vi "spiral scan.vi"(10 "maximum frequency":dbl, 11 "scan specification":T1) -> (0 "y":i16[](array[numeric]), 1 "x":i16[](array[numeric]), 2 "scan locations":u32[](array[numeric]), 3 "scan specification out":T1)   [LabVIEW 2010]
uses:
  scan_specification_tagResonant.ctl
  <vilib>/Analysis/NI_AALBase.lvlib
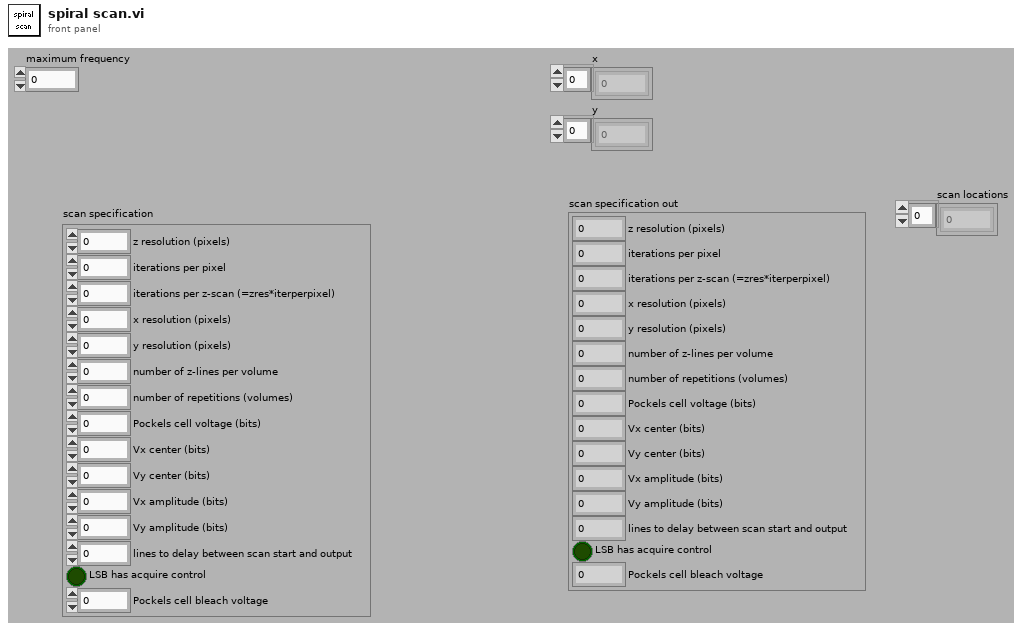
[diagram p1: front panel]
types:
  T1 = typedef "scan_specification_tagResonant.ctl" = cluster{"z resolution (pixels)":u16, "iterations per pixel":u16, "iterations per z-scan (=zres*iterperpixel)":u16, "x resolution (pixels)":u16, "y resolution (pixels)":u16, "number of z-lines per volume":u16, "number of repetitions (volumes)":i32, "Pockels cell voltage (bits)":i16, "Vx center (bits)":i16, "Vy center (bits)":i16, "Vx amplitude (bits)":i16, "Vy amplitude (bits)":i16, "lines to delay between scan start and output":u16, "LSB has acquire control":bool, "Pockels cell bleach voltage":i16}
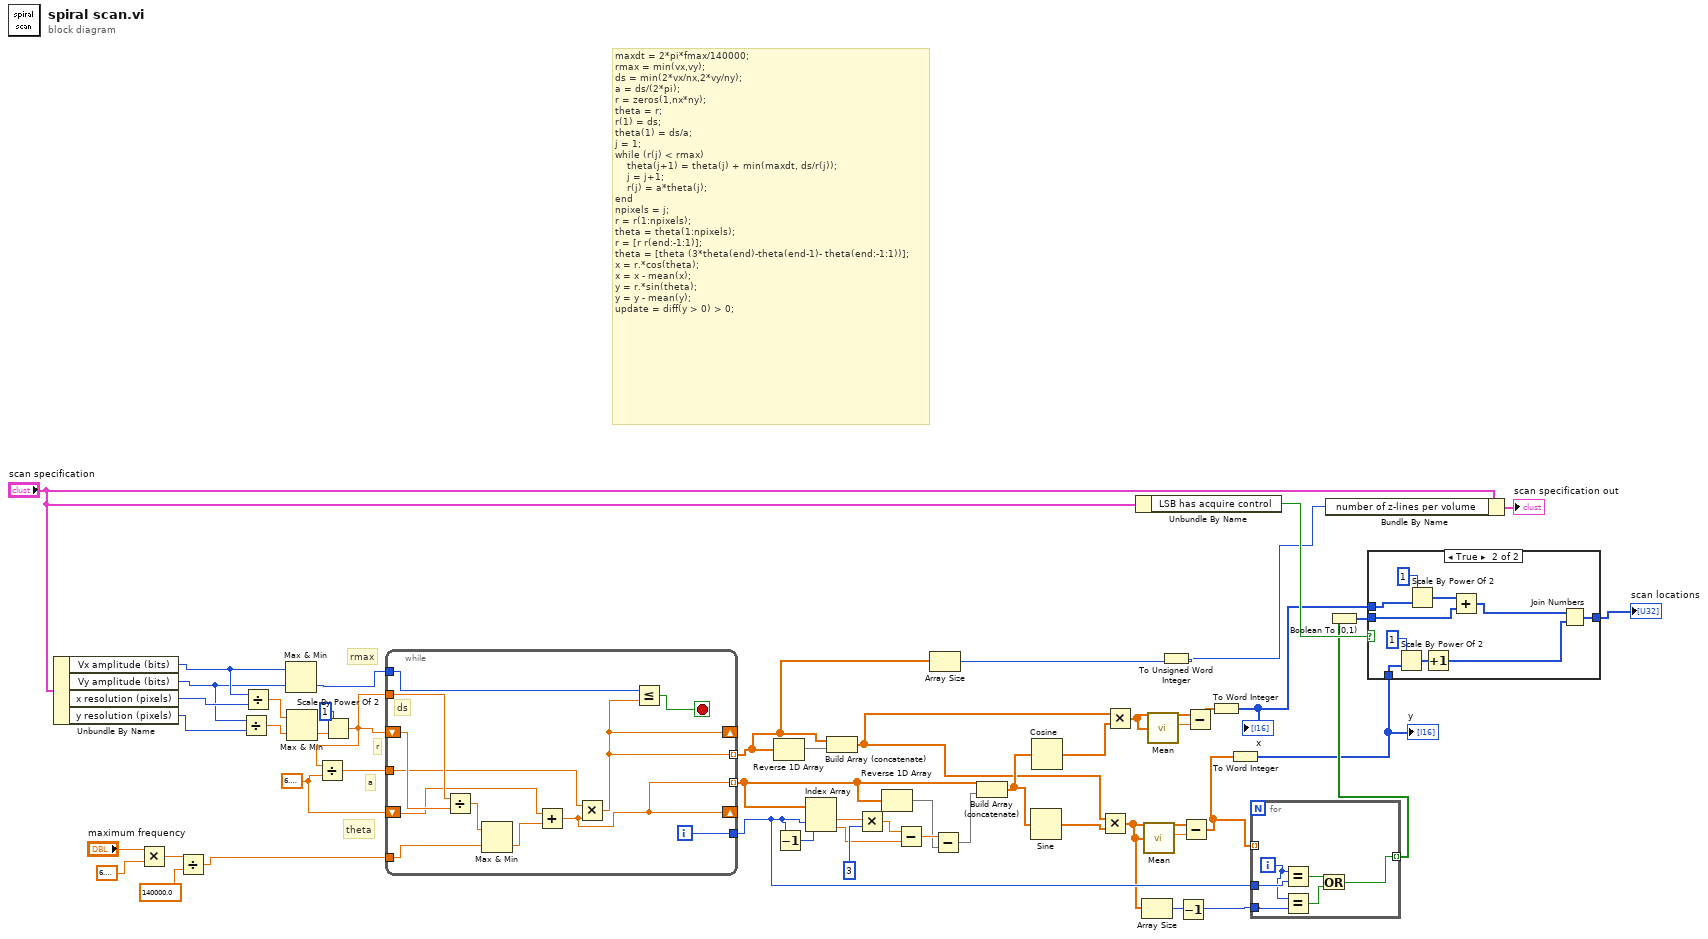
[diagram p0: block diagram]
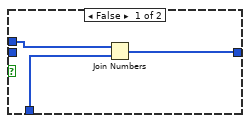
[diagram p2: hidden frame]
diagram:
  w40 = 6.283185307179586
  # "maxdt = 2*pi*fmax/140000;\nrmax = min(vx,vy);\nds = min(2*vx/nx,2*vy/ny);\na = ds/(2*pi);\nr = zeros(1,nx*ny);\ntheta = r;\nr(1) = ds;\ntheta(1) = ds/a;\nj = 1;\nwhile (r(j) < rmax)\n    theta(j+1) = theta(j) + min(maxdt, ds/r(j));\n    j = j+1;\n    r(j) = a*theta(j);\nend\nnpixels = j;\nr = r(1:npixels);\ntheta = theta(1:npixels);\nr = [r r(end:-1:1)];\ntheta = [theta (3*theta(end)-theta(end-1)- theta(end:-1:1))];\nx = r.*cos(theta);\nx = x - mean(x);\ny = r.*sin(theta);\ny = y - mean(y);\nupdate = diff(y > 0) > 0;"
  # "theta"
  # "a"
  # "r"
  # "rmax"
  n1 = Unbundle By Name("scan specification") -> ("Vx amplitude (bits)"=w49:i16, "Vy amplitude (bits)"=w47:i16, "x resolution (pixels)"=w48:u16, "y resolution (pixels)"=w46:u16)
  n2 = Multiply(x="maximum frequency", y=6.283185307179586) -> (x*y=w36:dbl)
  n3 = Divide(x=w36, y=140000.0) -> (x/y=w34:dbl)
  n4 = Divide(x=w47, y=w46) -> (x/y=w44:dbl)
  n5 = Divide(x=w49, y=w48) -> (x/y=w45:dbl)
  n6 = Max & Min(x=w49, y=w47) -> (min(x,y)=w37:i16)  [unwired: 1 out]
  n7 = Max & Min(x=w45, y=w44) -> (min(x,y)=w42:dbl)  [unwired: 1 out]
  n8 = Scale By Power Of 2(n=1, x=w42) -> (x*2^n=w11:dbl)
  n9 = Divide(x=w11, y=w40) -> (x/y=w41:dbl)
  n10 = while {
    shift-right: [w55] -> _
    shift-left: w11 -> [w61]
    tunnel: w11 -> [w62]
    tunnel: w41 -> [w58]
    shift-right: [w54] -> _
    shift-left: w40 -> [w59]
    tunnel: w37 -> [w57]
    tunnel: w34 -> [w63]
    tunnel: [w55] -> w12 mode=indexing
    tunnel: [w54] -> w25 mode=indexing
    tunnel: [w53] -> w4
    i -> [w53]
    stop <- w56 stop-if-true
    # "ds"
    n11 = Divide(x=w62, y=w61) -> (x/y=w60:dbl)
    n12 = Max & Min(x=w60, y=w63) -> (min(x,y)=w52:dbl)  [unwired: 1 out]
    n13 = Add(x=w59, y=w52) -> (x+y=w54:dbl)
    n14 = Multiply(x=w58, y=w54) -> (x*y=w55:dbl)
    n15 = Less Or Equal?(x=w57, y=w55) -> (x <= y?=w56:bool)
  }
  n16 = Reverse 1D Array(array=w12) -> (reversed array=w27:dbl[])
  n17 = Decrement(x=w4) -> (x-1=w5:i32)
  n18 = Index Array(array=w25, index #1=w4, index #2=w5) -> (element #1=w33:dbl, element #2=w30:dbl)
  n19 = Build Array (concatenate)(w12, w27) -> (w21:dbl[])
  n20 = Multiply(x=w33, y=3) -> (x*y=w31:dbl)
  n21 = Reverse 1D Array(array=w25) -> (reversed array=w28:dbl[])
  n22 = Subtract(x=w31, y=w30) -> (x-y=w29:dbl)
  n23 = Array Size(array=w12) -> (size(s)=w20:i32)
  n24 = Subtract(x=w29, y=w28) -> (x-y=w26:dbl[])
  n25 = Build Array (concatenate)(w25, w26) -> (w24:dbl[])
  n26 = Sine(x=w24) -> (sin(x)=w22:dbl[])
  n27 = Cosine(x=w24) -> (cos(x)=w23:dbl[])
  n28 = Multiply(x=w21, y=w22) -> (x*y=w3:dbl[])
  n29 = Multiply(x=w21, y=w23) -> (x*y=w9:dbl[])
  n30 = Unbundle By Name("scan specification") -> ("LSB has acquire control"=w51:bool)
  n31 = Array Size(array=w3) -> (size(s)=w2:i32)
  n32 = call <vilib>:"Mean.vi"("X"=w3) -> ("mean"=w7:dbl)  [unwired: 1 out]
  n33 = call <vilib>:"Mean.vi"("X"=w9) -> ("mean"=w8:dbl)  [unwired: 1 out]
  n34 = To Unsigned Word Integer(number=w20) -> (unsigned 16bit integer=w14:u16)
  n35 = Decrement(x=w2) -> (x-1=w1:i32)
  n36 = Subtract(x=w3, y=w7) -> (x-y=w6:dbl[])
  n37 = Subtract(x=w9, y=w8) -> (x-y=w10:dbl[])
  n38 = To Word Integer(number=w10) -> (16bit integer=w15:i16[])
  "x" <- w15
  n39 = To Word Integer(number=w6) -> (16bit integer=w16:i16[])
  "y" <- w16
  n40 = for {
    tunnel: w6 -> [_] mode=indexing
    tunnel: [w64] -> w19 mode=indexing
    tunnel: w4 -> [w69]
    tunnel: w1 -> [w66]
    i -> [w67]
    n41 = Equal?(x=w67, y=w69) -> (x = y?=w68:bool)
    n42 = Equal?(x=w67, y=w66) -> (x = y?=w65:bool)
    n43 = Or(x=w68, y=w65) -> (x .or. y?=w64:bool)
  }
  n44 = Bundle By Name(cluster="scan specification", "number of z-lines per volume"=w14) -> (→"scan specification out":T1)
  n45 = Boolean To (0,1)(Boolean=w19) -> (0, 1=w17:i16[])
  n46 = case shown="True" w51 {
    tunnel: w15 -> [w72 w78]
    tunnel: w16 -> [w71 w82]
    tunnel: [w70 w76] -> w13
    tunnel: w17 -> [_ w74]
    frame False {
      n47 = Join Numbers(hi=w72, lo=w71) -> ((hi.lo)=w70:u32[])
    }
    frame True {
      n48 = Scale By Power Of 2(n=1, x=w82) -> (x*2^n=w80:i16[])
      n49 = Scale By Power Of 2(n=1, x=w78) -> (x*2^n=w75:i16[])
      n50 = Increment(x=w80) -> (x+1=w77:i16[])
      n51 = Add(x=w75, y=w74) -> (x+y=w73:i16[])
      n52 = Join Numbers(hi=w73, lo=w77) -> ((hi.lo)=w76:u32[])
    }
  }
  "scan locations" <- w13
